vi "Read.vi"(8 "error in (no error)":errorcluster caption="错误输入（无错误）", 11 "Serial 输入":refnum<class "Serial.lvclass"> caption="DNL_LabVIEW Object in") -> (0 "error out":errorcluster caption="错误输出", 1 "ReadLength":i32, 2 "ReadBuf":string, 3 "Serial 输出":refnum<class "Serial.lvclass"> caption="DNL_LabVIEW Object out")   [LabVIEW 2012, in "Serial.lvclass"]
uses:
  Serial.lvclass
  PComm/PCOMM.lvlib
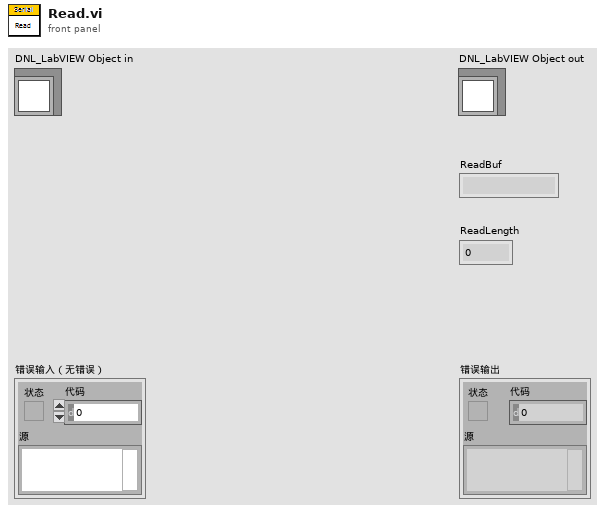
[diagram p1: front panel]
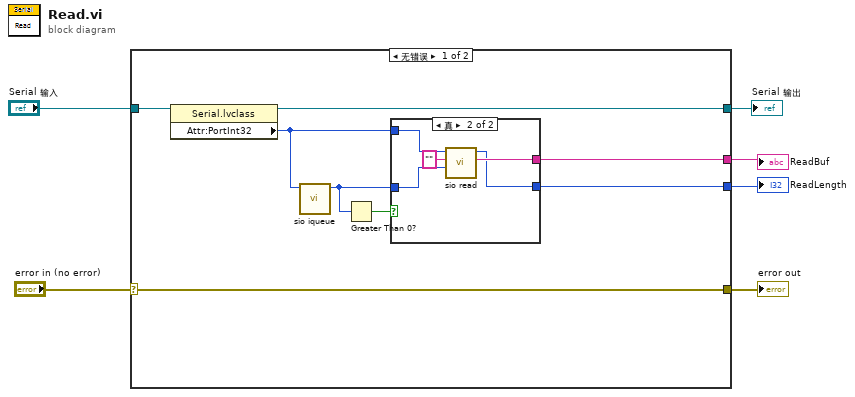
[diagram p0: block diagram]
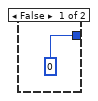
[diagram p2: hidden frame]
diagram:
  n1 = case shown="无错误" "error in (no error)" {
    selector: "error in (no error)" -> [w7 w22]
    tunnel: [w7 w22] -> w5
    tunnel: [w10 w21] -> w3
    tunnel: "Serial 输入" -> [w14 w21]
    tunnel: [w9 _] -> w2
    tunnel: [w8 _] -> w1
    frame No Error {
      n2 = property class="Serial.lvclass"(reference=w14) -> (reference out=w10:refnum<class "Serial.lvclass">, "Attr:PortInt32"=w13:i32)  [unwired: 1 in, 1 out]
      n3 = call "sio iqueue.vi"("port"=w13) -> ("function return"=w11:i32)  [unwired: 10 in]
      n4 = Greater Than 0?(x=w11) -> (x > 0?=w12:bool)
      n5 = case shown="真" w12 {
        tunnel: w13 -> [_ w20]
        tunnel: w11 -> [_ w17]
        tunnel: [_ w18] -> w9
        tunnel: [0 w16] -> w8
        frame False {
        }
        frame True {
          n6 = call "sio read.vi"("len"=w17, "buf"="", "port"=w20) -> ("buf out"=w18:string, "function return"=w16:i32)  [unwired: 7 in]
        }
      }
    }
    frame Error {
    }
  }
  "error out" <- w5
  "Serial 输出" <- w3
  "ReadBuf" <- w2
  "ReadLength" <- w1
